vi "UMLEditor InsertClassRefInAttribute.vi"(0 "AttributeIn":string, 1 "CompAgg":path[](array[path]), 5 "error in (no error)":errorcluster) -> (14 "AttributeOut":string, 19 "error out":errorcluster)   [LabVIEW 2016]
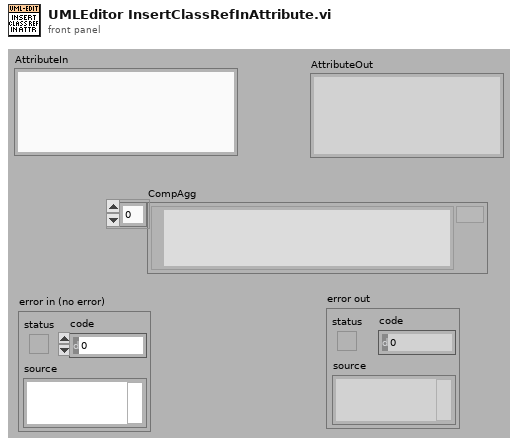
[diagram p1: front panel]
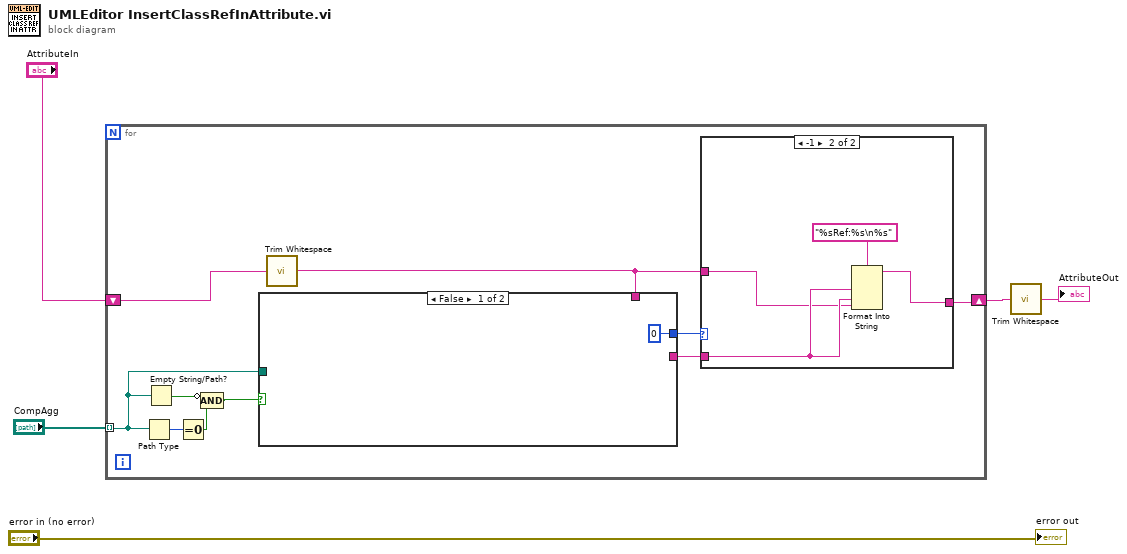
[diagram p0: block diagram]
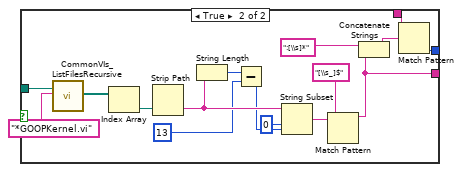
[diagram p2: hidden frame]
diagram:
  n1 = for {
    tunnel: "CompAgg" -> [w9] mode=indexing
    shift-right: [w14] -> w2
    shift-left: "AttributeIn" -> [w12]
    n2 = Path Type(1:w9) -> (0:w10:i16)
    n3 = Empty String/Path?(string/path=w9) -> (empty?=w8:bool)
    n4 = Equal To 0?(x=w10) -> (x = 0?=w7:bool)
    n5 = Compound Arithmetic op=AND(invert w8, w7) -> (w6:bool)
    n6 = call <vilib>:"Trim Whitespace.vi"("string"=w12) -> ("trimmed string"=w11:string)  [unwired: 1 in]
    n7 = case shown="False" w6 {
      tunnel: [0 ("offset past match") w26] -> w15
      tunnel: [_ w20] -> w13
      tunnel: w11 -> [_ w18]
      tunnel: w9 -> [_ w17]
      frame False {
      }
      frame True {
        n8 = call <resource>:"CommonVIs_ListFilesRecursive.vi"("directory path"=w17, "FileSearchPattern"="*GOOPKernel.vi") -> ("Files"=w31:path[])  [unwired: 4 in, 13 out]
        n9 = Index Array(array=w31) -> (element=w30:path)  [unwired: 1 in]
        n10 = Strip Path(path=w30) -> (name=w25:string)  [unwired: 1 out]
        n11 = String Length(string=w25) -> (length=w24:i32)
        n12 = Subtract(x=w24, y=13 ("length (rest)")) -> (x-y=w22:i32)
        n13 = String Subset(string=w25, offset (0)=0, length (rest)=w22) -> (substring=w21:string)
        n14 = Match Pattern(string=w21, regular expression="[\\s_]$") -> (before substring=w20:string)  [unwired: 4 out]
        n15 = Concatenate Strings(":[\\s]*" ("string"), w20) -> (w27:string)
        n16 = Match Pattern(string=w18, regular expression=w27) -> (offset past match=w26:i32)  [unwired: 4 out]
      }
    }
    n17 = case shown="-1" w15 {
      tunnel: w11 -> [w33 w34]
      tunnel: [w33 w35] -> w14
      tunnel: w13 -> [_ w36]
      frame 0, Default {
      }
      frame -1 {
        n18 = Format Into String(format string="%sRef:%s\n%s", w36, w36, w34) -> (resulting string=w35:string)  [unwired: 2 in, 1 out]
      }
    }
  }
  n19 = call <vilib>:"Trim Whitespace.vi"("string"=w2) -> ("trimmed string"=→"AttributeOut":string)  [unwired: 1 in]
  "error out" <- "error in (no error)"
